vi "Get Request Type.vi"(8 "error in (no error)":errorcluster, 11 "CreateSceneCollection in":refnum<class "CreateSceneCollection.lvclass">) -> (0 "error out":errorcluster, 2 "Request Type":string, 3 "CreateSceneCollection out":refnum<class "CreateSceneCollection.lvclass">)   [LabVIEW 2022 SP3, in "obs-websocket-lv.lvlib" / "CreateSceneCollection.lvclass"]
uses:
  CreateSceneCollection.lvclass
  CreateSceneCollection.lvclass/CreateSceneCollection.ctl
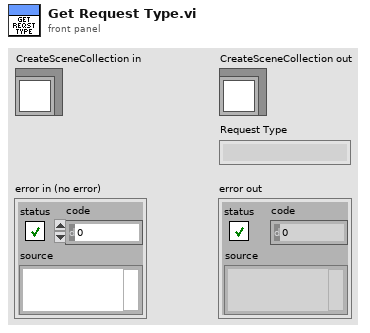
[diagram p1: front panel]
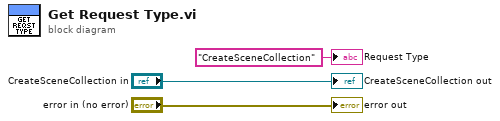
[diagram p0: block diagram]
diagram:
  "error out" <- "error in (no error)"
  "CreateSceneCollection out" <- "CreateSceneCollection in"
  "Request Type" <- "CreateSceneCollection" ("Request Type")
